vi "Main Page.vi"(8 "error in (no error)":errorcluster, 11 "Node Ptr":T1 format="%.0x") -> (0 "error out":errorcluster)   [LabVIEW 2019, in "Displacement Measurement CD System Explorer.lvlib"]
uses:
  Displacement Measurement CD System Explorer.lvlib
  <vilib>/NI VeriStand/Custom Device API/Custom Device Item Ref.ctl
  <vilib>/NI VeriStand/Custom Device API/Set Item Property (String).vi
  <vilib>/NI VeriStand/Custom Device API/Set Item Property (Double).vi
  <vilib>/NI VeriStand/Custom Device API/Custom Device API.lvlib
panel:
  in  "DAQmx Physical Channel":tag="PXI1Slot8/ai0:7"
  in  "Max. Voltage\n(V)":dbl=10.0
  in  "Min. Voltage\n(V)":dbl=-10.0
  in  "Sampling Frequency\n(S/Ch/s)":dbl=1000.0
  in  "Header":cluster{"Section Name":string}={"Section Name"="Custom Device Item Settings"}
  in  "Description":string
  in  "Name":string
  # "Device Configuration"
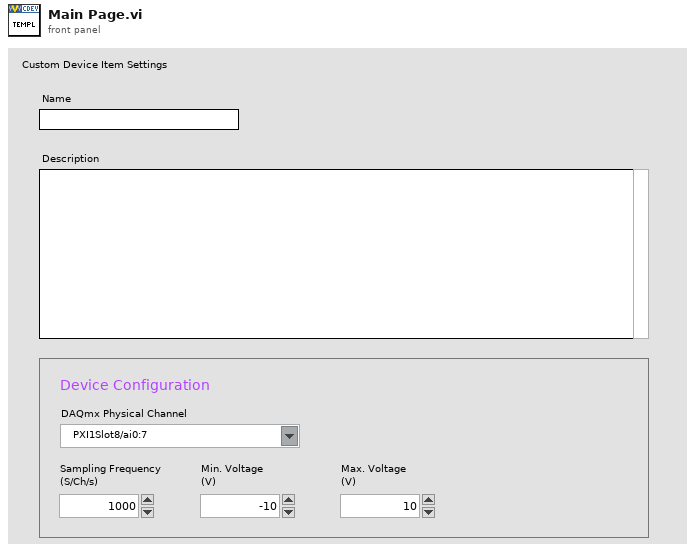
[diagram p1: front panel]
types:
  T1 = typedef "Custom Device API.lvlib/Custom Device Item Ref.ctl" = u64
  T2 = typedef "Custom Device API.lvlib/Custom Device Item Info.ctl" = cluster{"Name":string, "Is Channel":bool, "GUID":string, "Is Waveform":bool}
  T3 = typedef "Custom Device API.lvlib/Custom Device Commands.ctl" = enum16{"Default", "Item renamed", "Shutdown", "Dynamic button pressed"}
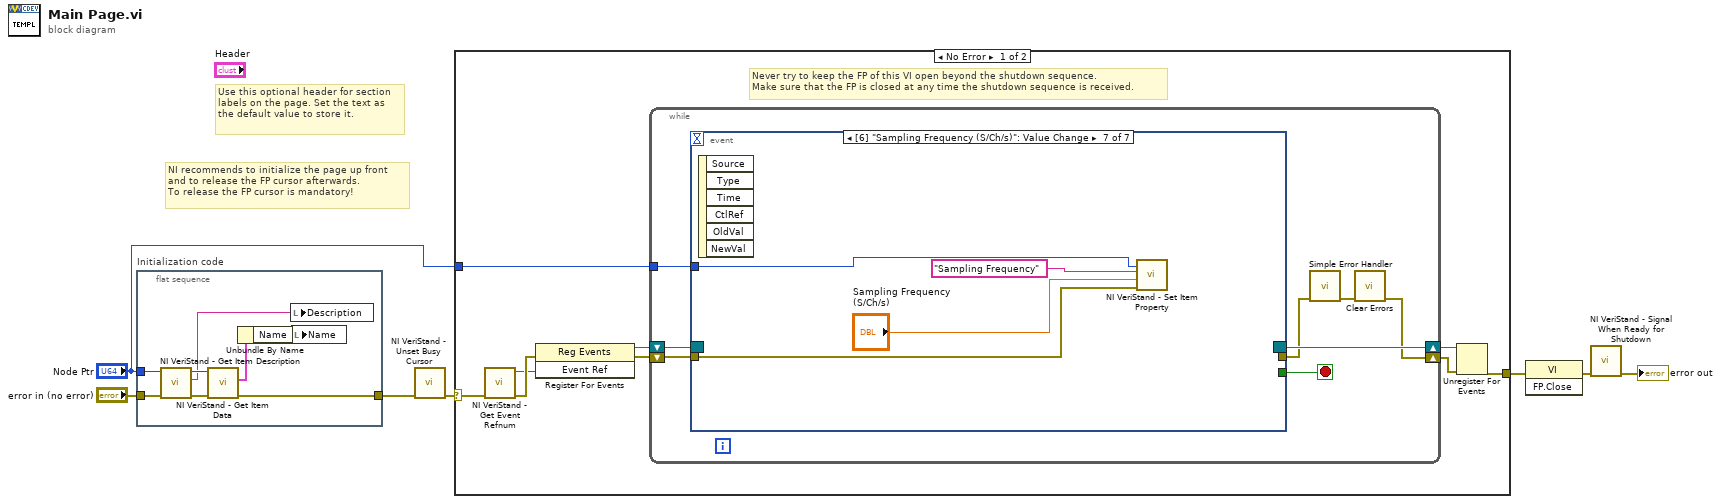
[diagram p0: block diagram]
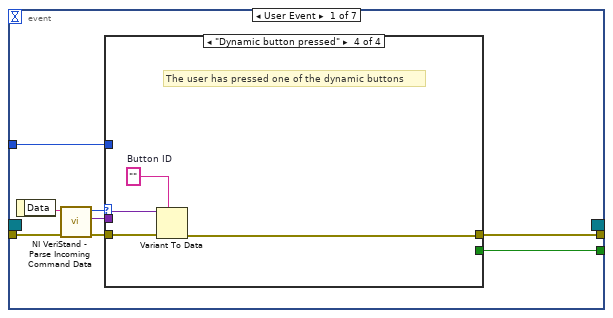
[diagram p2: hidden frame]
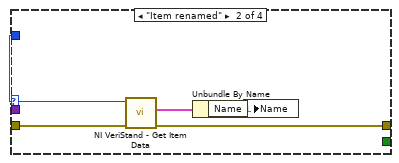
[diagram p4: hidden frame]
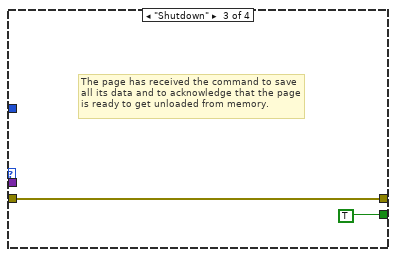
[diagram p5: hidden frame]
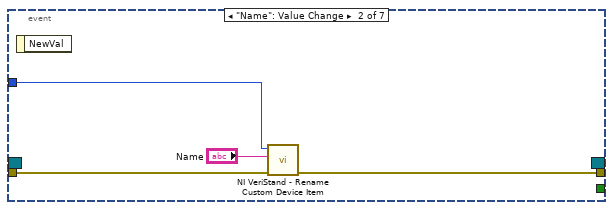
[diagram p6: hidden frame]
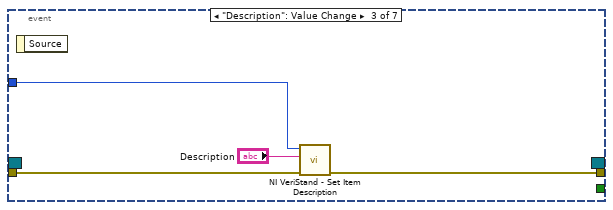
[diagram p7: hidden frame]
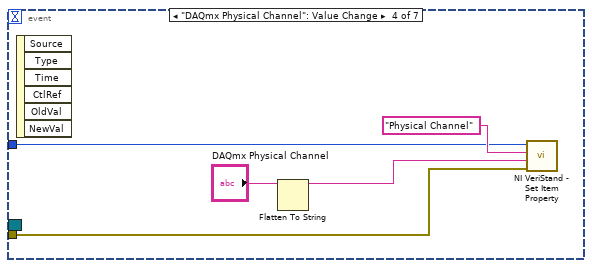
[diagram p8: hidden frame]
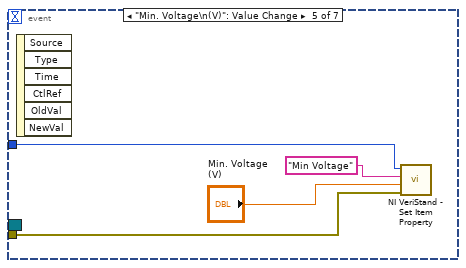
[diagram p9: hidden frame]
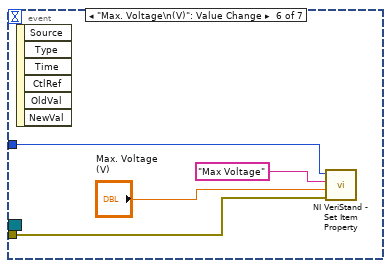
[diagram p10: hidden frame]
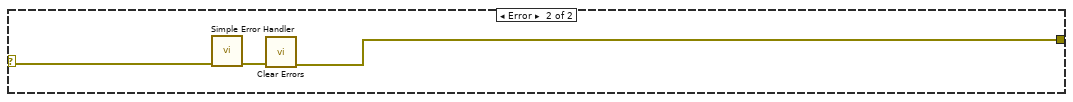
[diagram p11: hidden frame]
diagram:
  # "Use this optional header for section labels on the page. Set the text as the default value to store it."
  # "NI recommends to initialize the page up front\nand to release the FP cursor afterwards.\nTo release the FP cursor is mandatory!"
  n1 = flat-sequence "Initialization code" {
    tunnel: "error in (no error)" -> [w14]
    tunnel: "Node Ptr" -> [w13]
    tunnel: [w8] -> w4
    frame #0 {
      n2 = call <vilib>:"NI VeriStand - Get Item Description.vi"("error in (no error)"=w14, "Item Ref in"=w13) -> ("error out"=w11:errorcluster, "Description"=w12:string, "Item Ref out"=w15:T1)  [unwired: 7 out]
      n3 = call <vilib>:"NI VeriStand - Get Item Data.vi"("error in (no error)"=w11, "Item Ref in"=w15) -> ("error out"=w8:errorcluster, "Item Info"=w10:T2)  [unwired: 8 out]
      n4 = Unbundle By Name(w10) -> ("Name"=w9:string)
      n5 = local write "Description"(w12) -> ()
      n6 = local write "Name"(w9) -> ()
    }
  }
  n7 = call <vilib>:"NI VeriStand - Unset Busy Cursor.vi"("error in (no error)"=w4) -> ("error out"=w3:errorcluster)  [unwired: 10 out]
  n8 = case shown="No Error" w3 {
    selector: w3 -> [w16 w80]
    tunnel: [w21 w78] -> w7
    tunnel: "Node Ptr" -> [w17 _]
    frame No Error {
      # "Never try to keep the FP of this VI open beyond the shutdown sequence.\nMake sure that the FP is closed at any time the shutdown sequence is received."
      n9 = call <vilib>:"NI VeriStand - Get Event Refnum.vi"("error in (no error)"=w16) -> ("error out"=w24:errorcluster, "Event Ref"=w20:refnum<user-event>)  [unwired: 9 out]
      n10 = register-events(error in=w24, w20) -> (reference out=w18:refnum<event-registration>, error out=w19:errorcluster)  [unwired: 1 in]
      n11 = while {
        tunnel: w17 -> [w28]
        shift-right: [w25] -> w22
        shift-left: w19 -> [w31]
        shift-right: [w32] -> w23
        shift-left: w18 -> [w30]
        stop <- w29 stop-if-true
        n12 = event shown="[6] \"Sampling Frequency (S/Ch/s)\": Value Change" {
          selector: w30 -> [_ _ _ _ _ _ _]
          dyn-events: [_ _ _ _ _ _ _] -> w32
          timeout: _ -> [_ _ _ _ _ _ _]
          tunnel: w31 -> [w40 w56 w59 w62 w68 w72 w74]
          tunnel: [w36 _ _ _ _ _ _] -> w29
          tunnel: [w35 w55 w58 _ _ _ _] -> w27
          tunnel: w28 -> [w34 w54 w60 w61 w67 w71 w76]
          event User Event {
            n13 = event-data() -> ("Data"=w39:string)  [unwired: 1 out]
            n14 = call <vilib>:"NI VeriStand - Parse Incoming Command Data.vi"("error in (no error)"=w40, "Incoming data"=w39) -> ("error out"=w38:errorcluster, "Outgoing data"=w33:variant, "Action"=w37:T3)  [unwired: 7 out]
            n15 = case shown="\"Dynamic button pressed\"" w37 {
              tunnel: w38 -> [w41 w46 w47 w52]
              tunnel: [_ _ TRUE _] -> w36
              tunnel: [w41 w43 w47 w49] -> w35
              tunnel: w34 -> [_ w45 _ _]
              tunnel: w33 -> [_ _ _ w51]
              frame "Default", Default {
              }
              frame "Item renamed" {
                n16 = call <vilib>:"NI VeriStand - Get Item Data.vi"("error in (no error)"=w46, "Item Ref in"=w45) -> ("error out"=w43:errorcluster, "Item Info"=w44:T2)  [unwired: 8 out]
                n17 = Unbundle By Name(w44) -> ("Name"=w42:string)
                n18 = local write "Name"(w42) -> ()
              }
              frame "Shutdown" {
                # "The page has received the command to save all its data and to acknowledge that the page is ready to get unloaded from memory."
              }
              frame "Dynamic button pressed" {
                w50 = ""  # Button ID
                # "The user has pressed one of the dynamic buttons"
                n19 = Variant To Data(error in=w52, type=w50, Variant=w51) -> (error out=w49:errorcluster)  [unwired: 1 out]
              }
            }
          }
          event "Name": Value Change {
            n20 = event-data() -> ()  [unwired: 2 out]
            n21 = call <vilib>:"NI VeriStand - Rename Custom Device Item.vi"("error in (no error)"=w56, "New Name"="Name", "Item Ref in"=w54) -> ("error out"=w55:errorcluster)  [unwired: 1 in, 7 out]
          }
          event "Description": Value Change {
            n22 = event-data() -> ()  [unwired: 2 out]
            n23 = call <vilib>:"NI VeriStand - Set Item Description.vi"("error in (no error)"=w59, "Description"="Description", "Item Ref in"=w60) -> ("error out"=w58:errorcluster)  [unwired: 8 out]
          }
          event "DAQmx Physical Channel": Value Change {
            n24 = event-data() -> ()  [unwired: 7 out]
            n25 = Flatten To String(anything="DAQmx Physical Channel") -> (data string=w65:string)  [unwired: 3 in, 2 out]
            n26 = call-poly <vilib>:"NI VeriStand - Set Item Property.vi"("error in (no error)"=w62, "Value"=w65, "Property Name"="Physical Channel", "Item Ref in"=w61) -> ()  [unwired: 5 in, 3 out]
          }
          event "Min. Voltage\n(V)": Value Change {
            n27 = event-data() -> ()  [unwired: 7 out]
            n28 = call-poly <vilib>:"NI VeriStand - Set Item Property.vi"("error in (no error)"=w68, "Value"="Min. Voltage\n(V)", "Property Name"="Min Voltage", "Item Ref in"=w67) -> ()  [unwired: 5 in, 3 out]
          }
          event "Max. Voltage\n(V)": Value Change {
            n29 = event-data() -> ()  [unwired: 7 out]
            n30 = call-poly <vilib>:"NI VeriStand - Set Item Property.vi"("error in (no error)"=w72, "Value"="Max. Voltage\n(V)", "Property Name"="Max Voltage", "Item Ref in"=w71) -> ()  [unwired: 5 in, 3 out]
          }
          event "Sampling Frequency\n(S/Ch/s)": Value Change {
            n31 = event-data() -> ()  [unwired: 7 out]
            n32 = call-poly <vilib>:"NI VeriStand - Set Item Property.vi"("error in (no error)"=w74, "Value"="Sampling Frequency\n(S/Ch/s)", "Property Name"="Sampling Frequency", "Item Ref in"=w76) -> ()  [unwired: 5 in, 3 out]
          }
        }
        n33 = call <vilib>:"Simple Error Handler.vi"("error in (no error)"=w27) -> ("error out"=w26:errorcluster)  [unwired: 1 in, 7 out]
        n34 = call <vilib>:"Clear Errors.vi"("error in (no error)"=w26) -> ("error out"=w25:errorcluster)  [unwired: 1 in, 5 out]
      }
      n35 = Unregister For Events(event registration refnum=w23, error in=w22) -> (error out=w21:errorcluster)
    }
    frame Error {
      n36 = call <vilib>:"Simple Error Handler.vi"("error in (no error)"=w80) -> ("error out"=w79:errorcluster)  [unwired: 1 in, 7 out]
      n37 = call <vilib>:"Clear Errors.vi"("error in (no error)"=w79) -> ("error out"=w78:errorcluster)  [unwired: 1 in, 5 out]
    }
  }
  n38 = invoke class="VI" method="FP.Close"(error in=w7) -> (error out=w6:errorcluster)  [unwired: 2 in, 2 out]
  n39 = call <vilib>:"NI VeriStand - Signal When Ready for Shutdown.vi"("error in (no error)"=w6) -> ("error out"=→"error out":errorcluster)  [unwired: 10 out]
